vi "RP sweep skip old data.vi"(10 "First new data":i32, 11 "Input stream":i32[][](array[numeric])) -> (2 "Found":bool, 3 "Output stream":i32[][](array[numeric]))   [LabVIEW 2015]
panel:
  out "index of element":i32
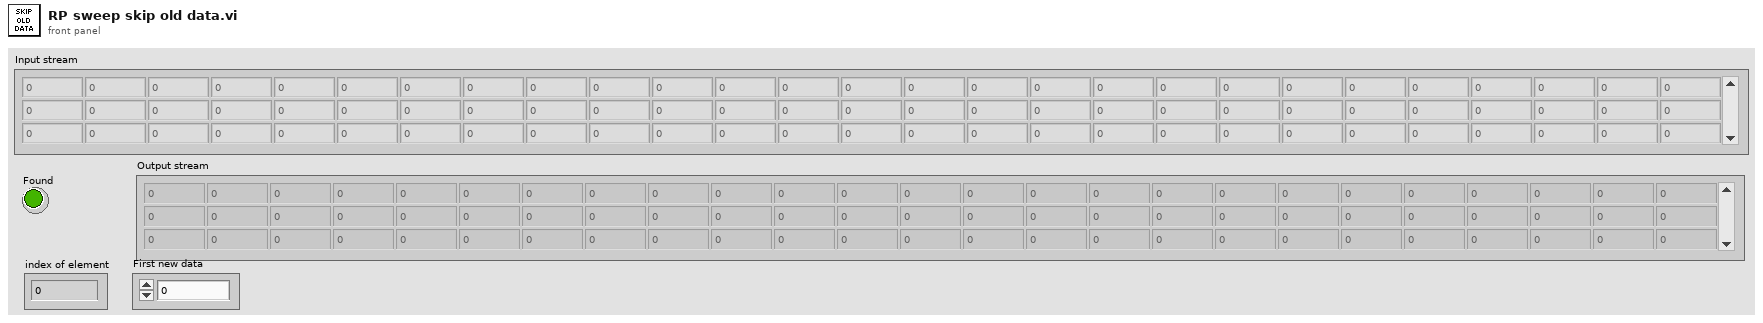
[diagram p1: front panel]
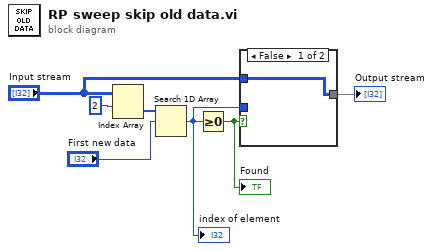
[diagram p0: block diagram]
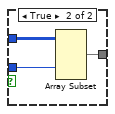
[diagram p2: hidden frame]
diagram:
  n1 = Index Array(array="Input stream", index (row)=2) -> (element=w1:i32[])  [unwired: 1 in]
  n2 = Search 1D Array(1D array=w1, element="First new data") -> (index of element=w3:i32)  [unwired: 1 in]
  "index of element" <- w3
  n3 = Greater Or Equal To 0?(x=w3) -> (x >= 0?=w5:bool)
  "Found" <- w5
  n4 = case shown="False" w5 {
    tunnel: "Input stream" -> [w8 w11]
    tunnel: w3 -> [_ w10]
    tunnel: [w8 w9] -> w2
    frame False {
    }
    frame True {
      n5 = Array Subset(array=w11, index (col)=w10) -> (w9:i32[][])  [unwired: 3 in]
    }
  }
  "Output stream" <- w2
